vi "USER_EDITOR_records_click_discard.vi"(10 "CellPosition":T2, 11 "event_structure_shift_register_in":T1={"REF_EDIT_clicked_row"=-1, "REF_EDIT_selected_row"=-1, "SQL_EDIT_clicked_row"=-1, "SQL_EDIT_selected_row"=-1, "ARCH_EDIT_selected_row"=-1, "ARCH_EDIT_clicked_row"=-1, "USER_EDIT_selected_row"=-1, "USER_EDIT_clicked_row"=-1, "REPORT_GEAR_toggle_all_results"=FALSE}) -> (2 "Discard?":bool, 3 "event_structure_shift_register_out":T1={"REF_EDIT_clicked_row"=-1, "REF_EDIT_selected_row"=-1, "SQL_EDIT_clicked_row"=-1, "SQL_EDIT_selected_row"=-1, "ARCH_EDIT_selected_row"=-1, "ARCH_EDIT_clicked_row"=-1, "USER_EDIT_selected_row"=-1, "USER_EDIT_clicked_row"=-1, "REPORT_GEAR_toggle_all_results"=FALSE})   [LabVIEW 2019]
uses:
  CLIENT_event_structure_shift_register.ctl
  <vilib>/Utility/miscctls.llb/LVRowAndColumnTypeDef.ctl
  FGV/USER_EDITOR_records_display/FGV_USER_EDITOR_records_display.ctl
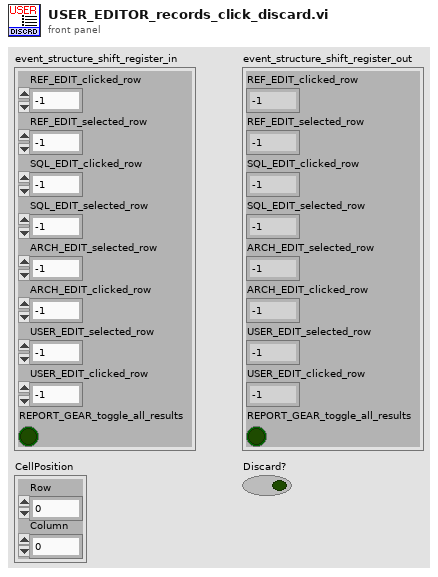
[diagram p1: front panel]
types:
  T1 = typedef "CLIENT_event_structure_shift_register.ctl" = cluster{"REF_EDIT_clicked_row":i32, "REF_EDIT_selected_row":i32, "SQL_EDIT_clicked_row":i32, "SQL_EDIT_selected_row":i32, "ARCH_EDIT_selected_row":i32, "ARCH_EDIT_clicked_row":i32, "USER_EDIT_selected_row":i32, "USER_EDIT_clicked_row":i32, "REPORT_GEAR_toggle_all_results":bool}
  T2 = typedef "LVRowAndColumnTypeDef.ctl" = cluster{"Row":i32, "Column":i32}
  T3 = typedef "FGV_USER_EDITOR_records_display.ctl" = enum16{"initialize", "set_user_edit_tables_names", "set_headers", "set_records", "get_user_edit_table_name", "get_user_edit_hist_table_name", "get_headers", "get_uneditable_columns", "get_all_info", "record_added?", "record_inserted?", "record_edited?", "record_updated?", "record_deleted?", "discard_changes"}
  T4 = typedef "USER_EDITOR_all_info.ctl" = cluster{"user_table":string, "user_history":string, "headers":string[], "uneditable_columns":string[], "uneditable_columns":i32[], "editable_columns":i32[], "values_in_database":string[][], "size":cluster{"columns":i32, "SQL_rows":i32, "disp_rows":i32}, "USER_record_states":T5[]}
  T5 = typedef "SQL_record_states.ctl" = enum16{"Equal", "Added", "Edited", "Deleted"}
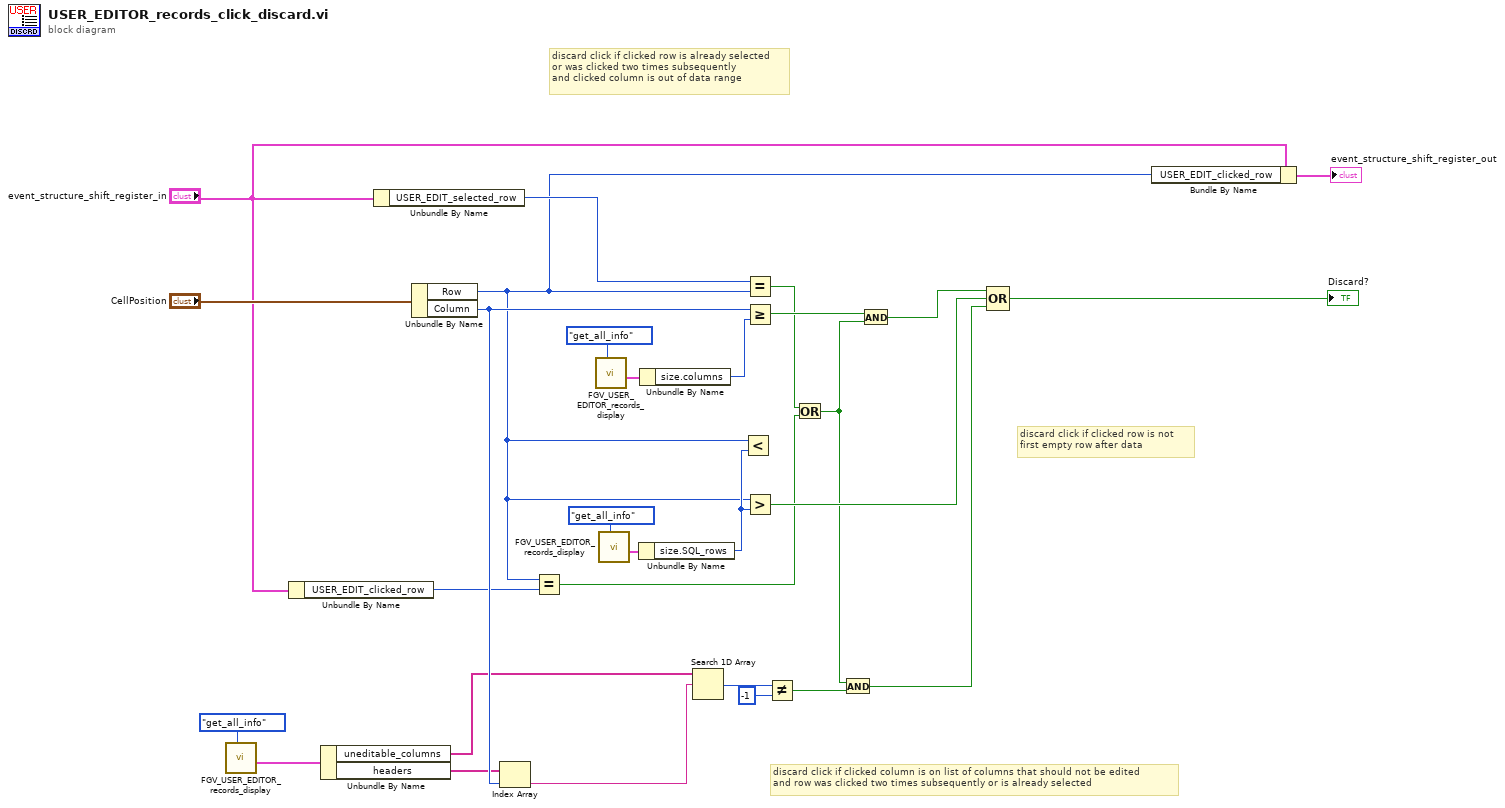
[diagram p0: block diagram]
diagram:
  # "discard click if clicked column is on list of columns that should not be edited\nand row was clicked two times subsequently or is already selected"
  # "discard click if clicked row is not \nfirst empty row after data"
  # "discard click if clicked row is already selected\nor was clicked two times subsequently\nand clicked column is out of data range"
  n1 = call "FGV_USER_EDITOR_records_display.vi"("options"=FGV_USER_EDITOR_records_display."get_all_info") -> ("all_info"=w4:T4)  [unwired: 7 in, 3 out]
  n2 = Unbundle By Name("event_structure_shift_register_in") -> ("USER_EDIT_clicked_row"=w13:i32)
  n3 = Unbundle By Name(w4) -> ("uneditable_columns"=w6:string[], "headers"=w7:string[])
  n4 = Unbundle By Name("event_structure_shift_register_in") -> ("USER_EDIT_selected_row"=w17:i32)
  n5 = Unbundle By Name("CellPosition") -> ("Row"=w12:i32, "Column"=w25:i32)
  n6 = Index Array(array=w7, index=w25) -> (element=w24:string)
  n7 = Equal?(x=w12, y=w13) -> (x = y?=w9:bool)
  n8 = call "FGV_USER_EDITOR_records_display.vi"("options"=FGV_USER_EDITOR_records_display."get_all_info") -> ("all_info"=w2:T4)  [unwired: 7 in, 3 out]
  n9 = call "FGV_USER_EDITOR_records_display.vi"("options"=FGV_USER_EDITOR_records_display."get_all_info") -> ("all_info"=w1:T4)  [unwired: 7 in, 3 out]
  n10 = Unbundle By Name(w1) -> ("size.SQL_rows"=w16:i32)
  n11 = Unbundle By Name(w2) -> ("size.columns"=w27:i32)
  n12 = Search 1D Array(1D array=w6, element=w24) -> (index of element=w23:i32)  [unwired: 1 in]
  n13 = Less?(x=w12, y=w16) -> ()  [unwired: 1 out]
  n14 = Equal?(x=w17, y=w12) -> (x = y?=w10:bool)
  n15 = Greater Or Equal?(x=w25, y=w27) -> (x >= y?=w11:bool)
  n16 = Greater?(x=w12, y=w16) -> (0:w18:bool)
  n17 = Not Equal?(x=w23, y=-1) -> (x != y?=w15:bool)
  n18 = Or(x=w10, y=w9) -> (x .or. y?=w8:bool)
  n19 = And(x=w8, y=w15) -> (x .and. y?=w20:bool)
  n20 = And(x=w11, y=w8) -> (x .and. y?=w21:bool)
  n21 = Compound Arithmetic op=OR(w21, w18, w20) -> (→"Discard?":bool)
  n22 = Bundle By Name(cluster="event_structure_shift_register_in", "USER_EDIT_clicked_row"=w12) -> (→"event_structure_shift_register_out":T1)
